vi "Convert To JSON Comp Format.vi"(11 "input settings":T2={"sample rate"=51200.0, "range"=5.0, "terminal configuration"=enum."Pseudodifferential"}) -> (3 "input settings JSON":T1={"sample rate"=51200.0, "range"=5.0, "terminal configuration"=""})   [LabVIEW 2021, in "Analog Input Settings.lvlib"]
uses:
  Analog Input Settings.lvlib
  service/generation/controls/analog input settings.ctl
  service/generation/controls/terminal configuration.ctl
  analog input settings_json.ctl
  service/generation/controls/AudioGenTypeDefs.lvlib
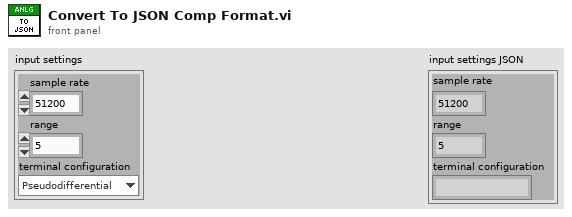
[diagram p1: front panel]
types:
  T1 = typedef "Analog Input Settings.lvlib/analog input settings_json.ctl" = cluster{"sample rate":dbl, "range":dbl, "terminal configuration":string}
  T2 = typedef "AudioGenTypeDefs.lvlib/analog input settings.ctl" = cluster{"sample rate":dbl, "range":dbl, "terminal configuration":T3}
  T3 = typedef "AudioGenTypeDefs.lvlib/terminal configuration.ctl" = enum32{"Default", "RSE", "Differential", "Pseudodifferential"}
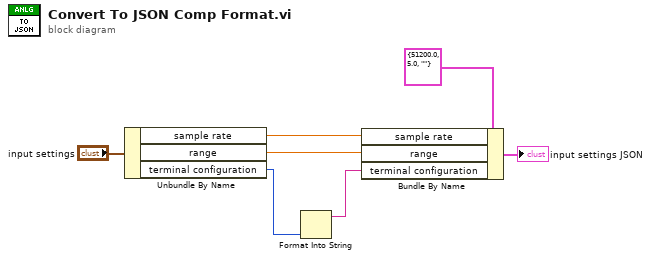
[diagram p0: block diagram]
diagram:
  n1 = Unbundle By Name("input settings") -> ("sample rate"=w6:dbl, "range"=w5:dbl, "terminal configuration"=w4:T3)
  n2 = Format Into String(w4) -> (resulting string=w3:string)  [unwired: 3 in, 1 out]
  n3 = Bundle By Name(cluster=T1 {"sample rate"=51200.0, "range"=5.0, "terminal configuration"=""} ("output settings JSON"), "sample rate"=w6, "range"=w5, "terminal configuration"=w3) -> (→"input settings JSON":T1)
